vi "ScanivalveClose.vi"(2 "error in (no error)":errorcluster, 3 "timeout ms (20000)":i32=20000, 5 "connection ID":refnum<k5>) -> (0 "error out":errorcluster)   [LabVIEW 2019]
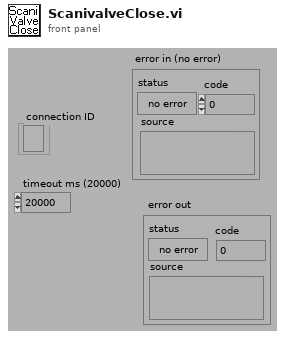
[diagram p1: front panel]
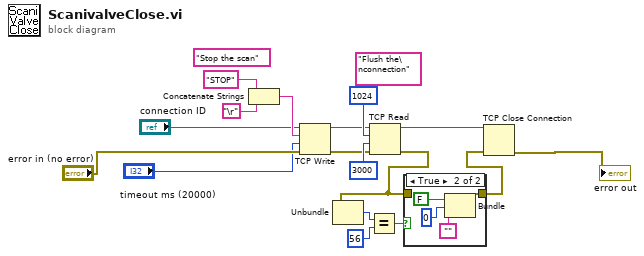
[diagram p0: block diagram]
diagram:
  (unwired) "Flush the\nconnection"
  (unwired) "Stop the scan"
  n1 = Concatenate Strings("STOP", "\r") -> (w2:string)
  n2 = TCP Write(connection ID="connection ID", data in=w2, error in (no error)="error in (no error)", 9:"timeout ms (20000)") -> (connection ID out=w5:refnum<k5>, error out=w6:errorcluster)  [unwired: 1 out]
  n3 = TCP Read(connection ID=w5, bytes to read=1024, error in (no error)=w6, 9:3000) -> (connection ID out=w7:refnum<k5>, error out=w13:errorcluster)  [unwired: 1 in, 1 out]
  n4 = Unbundle(w13) -> ("code"=w10:i32)  [unwired: 2 out]
  n5 = Equal?(x=w10, y=56) -> (x = y?=w12:bool)
  n6 = case shown="True" w12 {
    tunnel: [w18 w19] -> w14
    tunnel: w13 -> [w18 _]
    frame False {
    }
    frame True {
      n7 = Bundle(FALSE, 0, "") -> (w19:errorcluster)  [unwired: 1 in]
    }
  }
  n8 = TCP Close Connection(connection ID=w7, error in (no error)=w14) -> (error out=→"error out":errorcluster)  [unwired: 1 in, 1 out]
